vi "ReadCarexFile.vi"(6 "Line/(Circle)":enum16{"Circle", "Line"}(ring), 8 "error in (no error)":errorcluster, 10 "File Path":path, 11 "CarexData In":refnum<class "CarexMData.lvclass">) -> (0 "error out":errorcluster, 3 "CarexData Out":refnum<class "CarexMData.lvclass">)   [LabVIEW 2014]
uses:
  Dropbox/Research/LabView/CustomVI/CustomVI.lvlib
  <vilib>/Utility/file.llb/Read From Spreadsheet File (string).vi
  CarexMData.lvclass
panel:
  out "Multicolumn Listbox":i32(listbox)
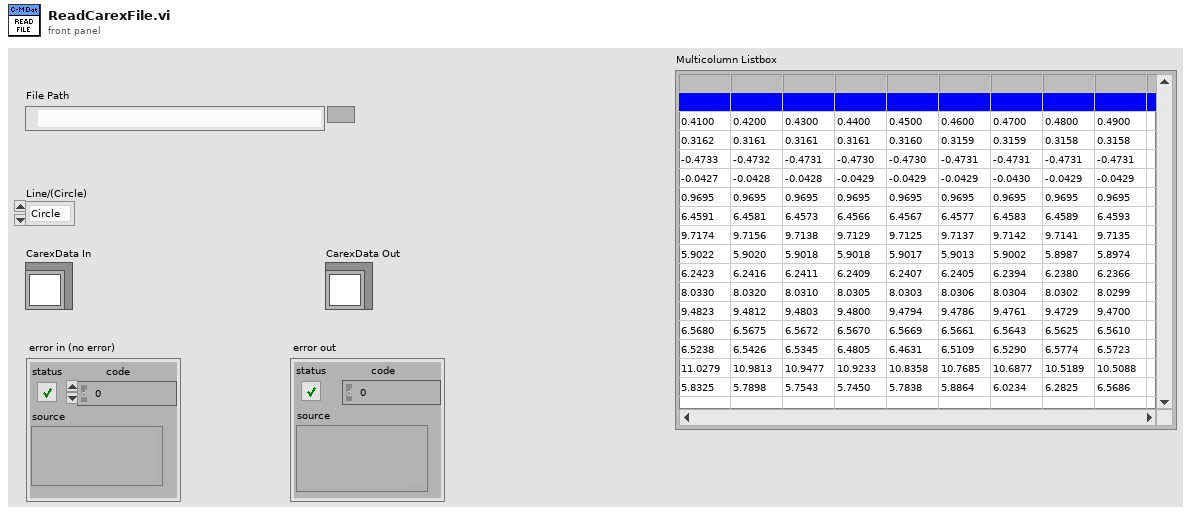
[diagram p1: front panel]
types:
  T1 = cluster{"Lines to Output":i32, "Total Lines to Read":i32}
  T2 = cluster{"MotorOn":bool, "EstGH":bool, "TensionMode":u16}
  T3 = cluster{"Total Lines to Read":i32, "Lines to Output":i32}
  T4 = cluster{"array type (2D Dbl)[0]":dbl, "array type (2D Dbl)[1]":dbl}
  T5 = cluster{"array type (2D Dbl)[0]":dbl, "array type (2D Dbl)[1]":dbl, "array type (2D Dbl)[2]":dbl, "array type (2D Dbl)[3]":dbl, "array type (2D Dbl)[4]":dbl, "array type (2D Dbl)[5]":dbl}
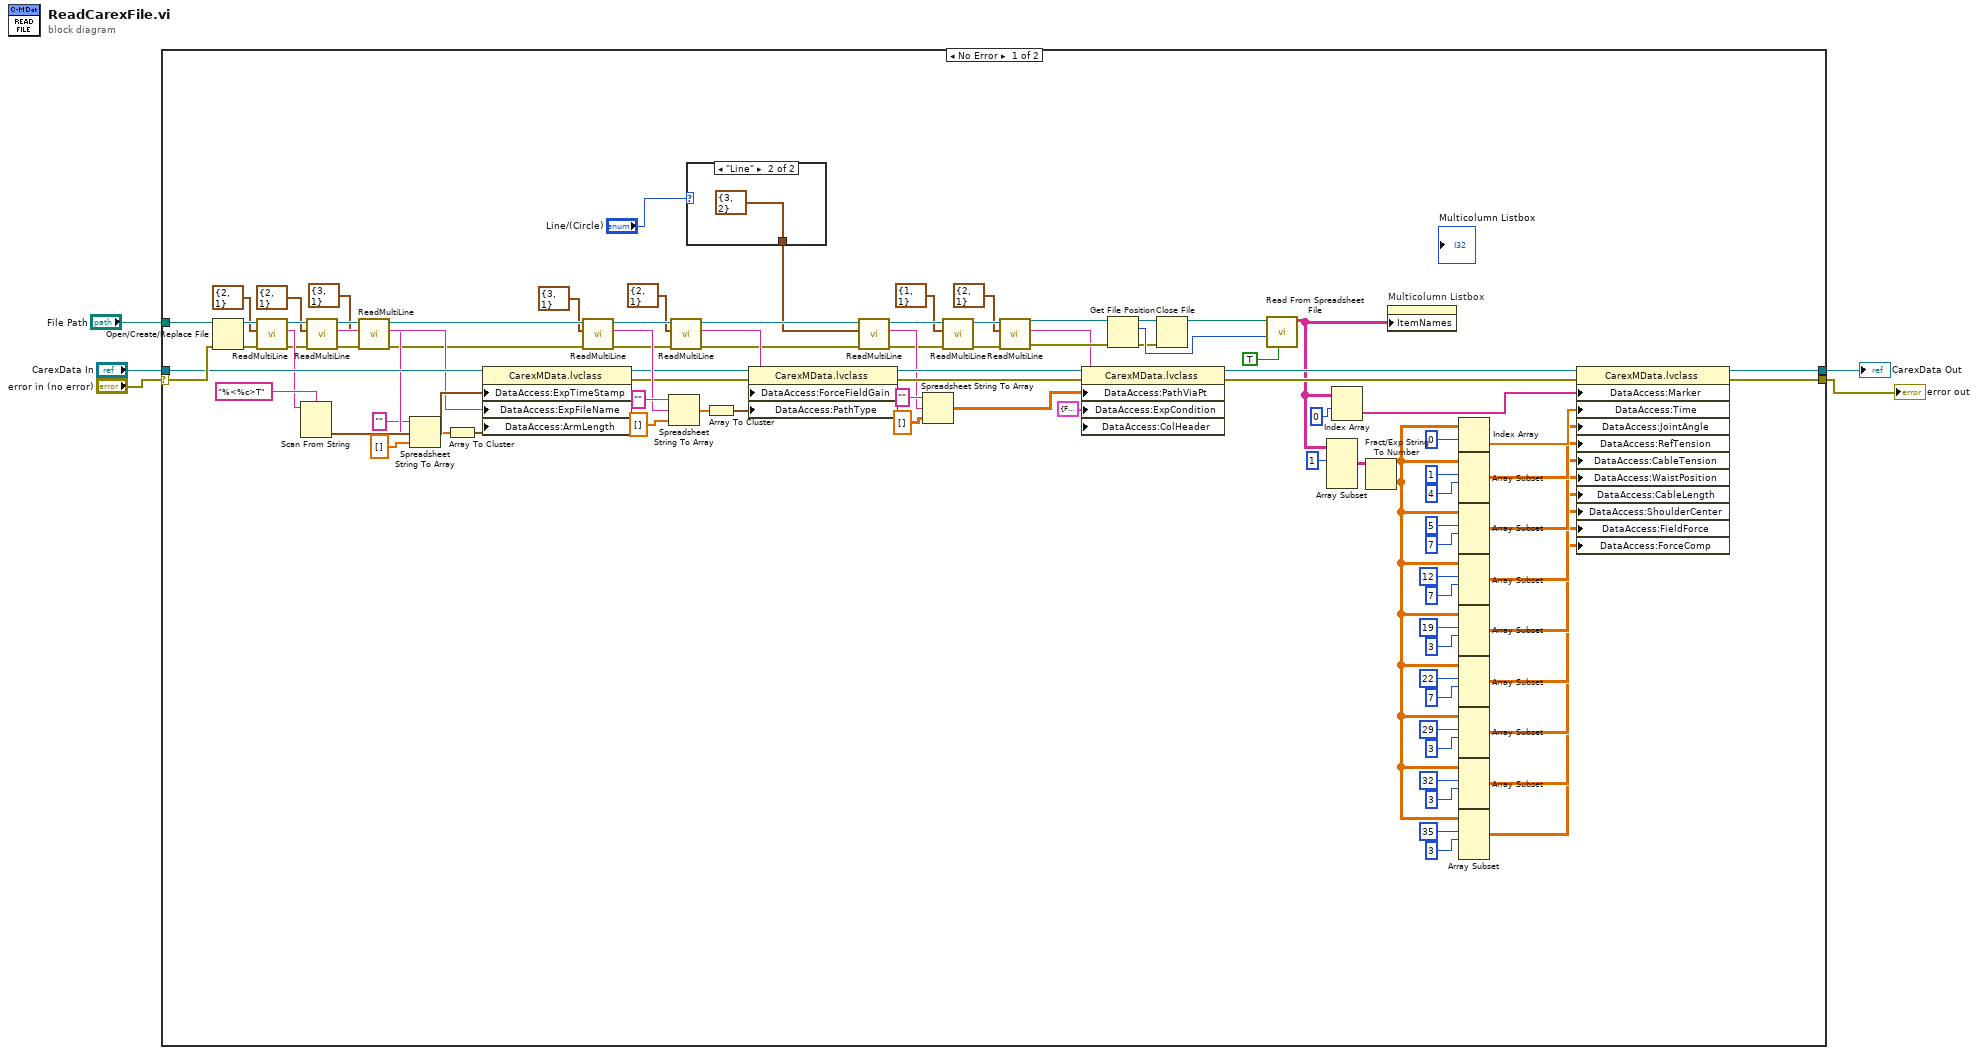
[diagram p0: block diagram]
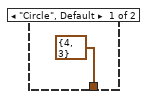
[diagram p2: hidden frame]
diagram:
  n1 = case shown="No Error" "error in (no error)" {
    selector: "error in (no error)" -> [w100 w105]
    tunnel: [w17 w104] -> w1
    tunnel: [w16 w105] -> w5
    tunnel: "File Path" -> [w101 _]
    tunnel: "CarexData In" -> [w98 w104]
    frame No Error {
      n2 = Open/Create/Replace File(file path (use dialog)=w101, error in=w100) -> (refnum out=w96:refnum<file>, error out=w95:errorcluster)  [unwired: 4 in, 1 out]
      n3 = call "ReadMultiLine.vi"("error in (no error)"=w95, "Lines to Read/Output"=T1 {"Lines to Output"=2, "Total Lines to Read"=1} ("Cluster"), "refnum in"=w96) -> ("error out"=w92:errorcluster, "Strings"=w94:string, "refnum out"=w93:refnum<file>)  [unwired: 6 in]
      n4 = Scan From String(format string="%<%c>T", input string=w94) -> (output 1=w97:timestamp)  [unwired: 3 in, 3 out]
      n5 = call "ReadMultiLine.vi"("error in (no error)"=w92, "Lines to Read/Output"=T1 {"Lines to Output"=2, "Total Lines to Read"=1} ("Cluster"), "refnum in"=w93) -> ("error out"=w89:errorcluster, "Strings"=w91:string, "refnum out"=w90:refnum<file>)  [unwired: 6 in]
      n6 = call "ReadMultiLine.vi"("error in (no error)"=w89, "Lines to Read/Output"=T1 {"Lines to Output"=3, "Total Lines to Read"=1} ("Cluster"), "refnum in"=w90) -> ("error out"=w82:errorcluster, "Strings"=w88:string, "refnum out"=w83:refnum<file>)  [unwired: 6 in]
      n7 = Spreadsheet String To Array(format string="", spreadsheet string=w88, array type (2D Dbl)=dbl[] []) -> (array=w85:dbl[])  [unwired: 1 in]
      n8 = Array To Cluster(array=w85) -> (cluster=w84:T4)
      n9 = property class="CarexMData.lvclass"(reference=w98, "DataAccess:ExpTimeStamp"=w97, "DataAccess:ExpFileName"=w91, "DataAccess:ArmLength"=w84) -> (reference out=w73:refnum<class "CarexMData.lvclass">, error out=w72:errorcluster)  [unwired: 1 in]
      n10 = call "ReadMultiLine.vi"("error in (no error)"=w82, "Lines to Read/Output"=T3 {"Total Lines to Read"=3, "Lines to Output"=1} ("Cluster"), "refnum in"=w83) -> ("error out"=w69:errorcluster, "Strings"=w74:string, "refnum out"=w70:refnum<file>)  [unwired: 6 in]
      n11 = Spreadsheet String To Array(format string="", spreadsheet string=w74, array type (2D Dbl)=dbl[] []) -> (array=w77:dbl[])  [unwired: 1 in]
      n12 = call "ReadMultiLine.vi"("error in (no error)"=w69, "Lines to Read/Output"=T1 {"Lines to Output"=2, "Total Lines to Read"=1} ("Cluster"), "refnum in"=w70) -> ("error out"=w66:errorcluster, "Strings"=w67:string, "refnum out"=w65:refnum<file>)  [unwired: 6 in]
      n13 = case shown="\"Line\"" "Line/(Circle)" {
        tunnel: [T1 {"Lines to Output"=4, "Total Lines to Read"=3} ("Cluster") T1 {"Lines to Output"=3, "Total Lines to Read"=2} ("Cluster")] -> w6
        frame "Circle", Default {
        }
        frame "Line" {
        }
      }
      n14 = Array To Cluster(array=w77) -> (cluster=w71:T5)
      n15 = property class="CarexMData.lvclass"(reference=w73, error in=w72, "DataAccess:ForceFieldGain"=w71, "DataAccess:PathType"=w67) -> (reference out=w62:refnum<class "CarexMData.lvclass">, error out=w61:errorcluster)
      n16 = call "ReadMultiLine.vi"("error in (no error)"=w66, "Lines to Read/Output"=w6, "refnum in"=w65) -> ("error out"=w58:errorcluster, "Strings"=w60:string, "refnum out"=w57:refnum<file>)  [unwired: 6 in]
      n17 = Spreadsheet String To Array(format string="", spreadsheet string=w60, array type (2D Dbl)=dbl[][] []) -> (array=w59:dbl[][])  [unwired: 1 in]
      n18 = call "ReadMultiLine.vi"("error in (no error)"=w58, "Lines to Read/Output"=T1 {"Lines to Output"=1, "Total Lines to Read"=1} ("Cluster"), "refnum in"=w57) -> ("error out"=w54:errorcluster, "refnum out"=w53:refnum<file>)  [unwired: 6 in, 1 out]
      n19 = call "ReadMultiLine.vi"("error in (no error)"=w54, "Lines to Read/Output"=T1 {"Lines to Output"=2, "Total Lines to Read"=1} ("Cluster"), "refnum in"=w53) -> ("error out"=w50:errorcluster, "Strings"=w8:string, "refnum out"=w51:refnum<file>)  [unwired: 6 in]
      n20 = property class="CarexMData.lvclass"(reference=w62, error in=w61, "DataAccess:PathViaPt"=w59, "DataAccess:ExpCondition"=T2 {"MotorOn"=FALSE, "EstGH"=FALSE, "TensionMode"=0} ("ExpCondition"), "DataAccess:ColHeader"=w8) -> (reference out=w48:refnum<class "CarexMData.lvclass">, error out=w47:errorcluster)
      n21 = Get File Position(4:w50, 7:w51) -> (0:w9:errorcluster, 2:w49:i64, 3:w11:refnum<file>)
      n22 = Close File(refnum=w11, error in=w9) -> (path=w10:path)  [unwired: 1 out]
      n23 = call-poly <vilib>:"Read From Spreadsheet File.vi"("transpose (no:F)"=TRUE, "start of read offset (chars.:0)"=w49, "file path (dialog if empty)"=w10) -> ("all rows"=w15:string[][])  [unwired: 4 in, 4 out]
      n24 = Array Subset(array=w15, index (row)=1 ("index")) -> (w45:string[][])  [unwired: 3 in]
      n25 = Index Array(array=w15, index (row)=0 ("disabled index (col)")) -> (element=w46:string[])  [unwired: 1 in]
      n26 = Fract/Exp String To Number(string=w45) -> (number=w27:dbl[][])  [unwired: 3 in, 1 out]
      n27 = property on="Multicolumn Listbox" class="MCListbox (strict)"("ItemNames"=w15) -> ()  [unwired: 2 in, 2 out]
      n28 = Index Array(array=w27, index (row)=0 ("index")) -> (element=w26:dbl[])  [unwired: 1 in]
      n29 = Array Subset(array=w27, index (row)=1 ("index"), length (row)=4 ("length")) -> (w25:dbl[][])  [unwired: 2 in]
      n30 = Array Subset(array=w27, index (row)=5 ("index"), length (row)=7 ("length")) -> (w24:dbl[][])  [unwired: 2 in]
      n31 = Array Subset(array=w27, index (row)=12 ("index"), length (row)=7 ("length")) -> (w23:dbl[][])  [unwired: 2 in]
      n32 = Array Subset(array=w27, index (row)=19 ("index"), length (row)=3 ("length")) -> (w22:dbl[][])  [unwired: 2 in]
      n33 = Array Subset(array=w27, index (row)=22 ("index"), length (row)=7 ("length")) -> (w21:dbl[][])  [unwired: 2 in]
      n34 = Array Subset(array=w27, index (row)=29 ("index"), length (row)=3 ("length")) -> (w20:dbl[][])  [unwired: 2 in]
      n35 = Array Subset(array=w27, index (row)=32 ("index"), length (row)=3 ("length")) -> (w19:dbl[][])  [unwired: 2 in]
      n36 = Array Subset(array=w27, index (row)=35 ("index"), length (row)=3 ("length")) -> (w18:dbl[][])  [unwired: 2 in]
      n37 = property class="CarexMData.lvclass"(reference=w48, error in=w47, "DataAccess:Marker"=w46, "DataAccess:Time"=w26, "DataAccess:JointAngle"=w25, "DataAccess:RefTension"=w24, "DataAccess:CableTension"=w23, "DataAccess:WaistPosition"=w22, "DataAccess:CableLength"=w21, "DataAccess:ShoulderCenter"=w20, "DataAccess:FieldForce"=w19, "DataAccess:ForceComp"=w18) -> (reference out=w17:refnum<class "CarexMData.lvclass">, error out=w16:errorcluster)
    }
    frame Error {
    }
  }
  "CarexData Out" <- w1
  "error out" <- w5
